vi "Add New Pos.vi"(0 "CS++Motor in":refnum<class "CS++Motor.lvclass">, 1 "Referenced":bool[](array[boolean]), 3 "MovementList In":T2(array[cluster]), 4 "NewPos-Data":T1, 5 "error in (no error)":errorcluster, 7 "LastPos In":cluster{dbl[]}[](array[cluster]), 8 "Axis Overwrite?":bool, 9 "AxisNumber":u8, 11 "ActPos":dbl[](array[numeric])) -> (13 "LastPos Out":cluster{dbl[]}[](array[cluster]), 14 "CS++Motor out":refnum<class "CS++Motor.lvclass">, 17 "MovementList Out":T2(array[cluster]), 19 "error out":errorcluster)   [LabVIEW 2016, in "CS++Motor.lvlib" / "CS++Motor.lvclass"]
doc: "This VI adds new position information to the Motor Base class actor. This information is written in a list and the commands are sent to the device once it is not busy."
uses:
  CS++Motor.lvclass
  PV-Enum-n.ctl
  CSPP_Core/Classes/CS++ProcessVariables/ProcessVariable/PV.lvclass
  CS++Motor.lvclass/CS++Motor.ctl
  CSPP_Core/Classes/CS++ProcessVariables/ProcessVariable/PV.lvclass/PV.ctl
  CSPP_Core/Classes/CS++ProcessVariables/ProcessVariable/Write Data.vi
  CSPP_Core/Classes/CS++ProcessVariables/ProcessVariable/Write Timestamp.vi
  CSPP_Core/Classes/CS++ProcessVariables/ProcessVariable/Write Quality.vi
  CSPP_Core/Classes/CS++ProcessVariables/ProcessVariable/Write status.vi
  CSPP_Core/Classes/CS++ProcessVariables/PVConnection/PVConnection.lvclass
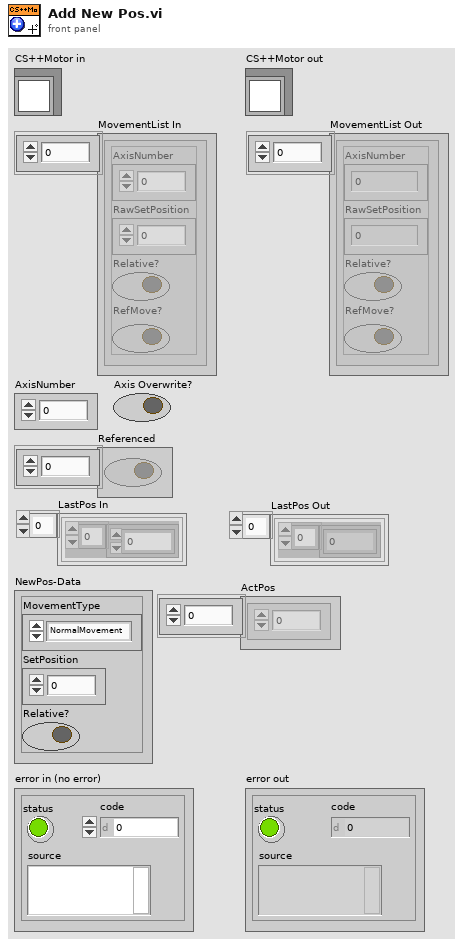
[diagram p1: front panel]
types:
  T1 = cluster{"MovementType":enum16{"NormalMovement", "ReferenceMovement", "StopMovement"}, "SetPosition":dbl, "Relative?":bool}
  T2 = cluster{"AxisNumber":u8, "RawSetPosition":dbl, "Relative?":bool, "RefMove?":bool}[]
  T3 = typedef "CS++Motor.lvlib/CS++Motor.lvclass/PV-Enum-n.ctl" = enum16{"PhysicalName", "unit", "ActPosition", "SetPosition", "RawSetPosition", "StartVelocity", "StopVelocity", "Acceleration", "RangeMin", "RangeMax", "Scaling", "ScalingOffset", "RangeRefError", "LogicalPositionArray", "NoOfCommands"}
  T4 = enum16{"NormalMovement", "ReferenceMovement", "StopMovement"}
  T5 = cluster{"AxisNumber":u8, "RawSetPosition":dbl, "Relative?":bool, "RefMove?":bool}
  T6 = cluster{"LogicalName":string, "PhysicalName":string, "unit":string, "Scaling":dbl, "Scaling Offset":dbl, "StartVelocity":dbl, "StopVelocity":dbl, "Acceleration":dbl, "RangeMin":dbl, "RangeMax":dbl, "LogicalPos-Array":cluster{"LogicalPosition":string, "SetPosition":dbl}[]}[]
  T7 = cluster{"LogicalName":string, "PhysicalName":string, "unit":string, "Scaling":dbl, "Scaling Offset":dbl, "StartVelocity":dbl, "StopVelocity":dbl, "Acceleration":dbl, "RangeMin":dbl, "RangeMax":dbl, "LogicalPos-Array":cluster{"LogicalPosition":string, "SetPosition":dbl}[]}
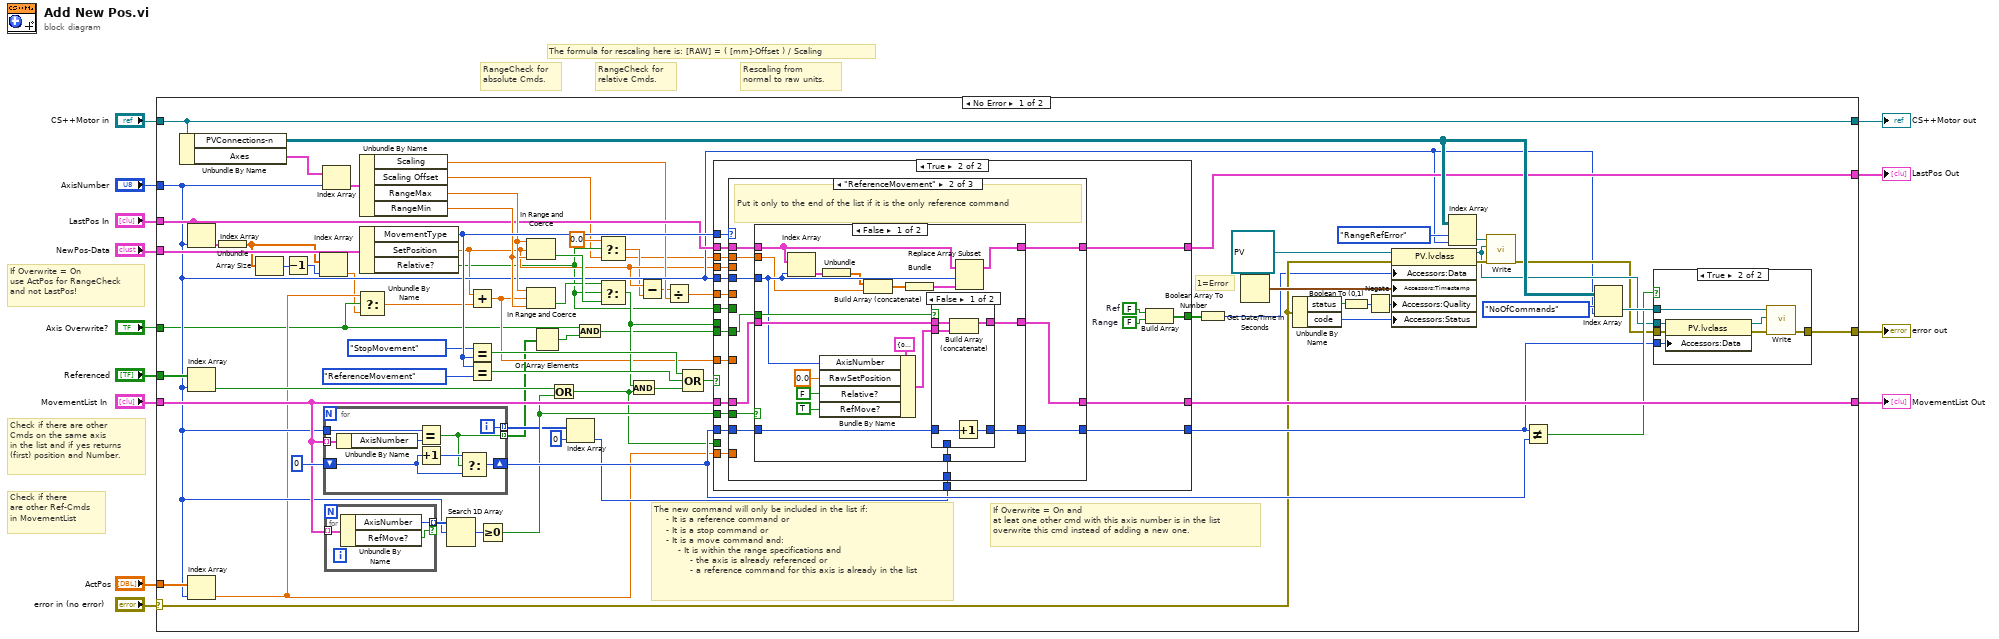
[diagram p0: block diagram]
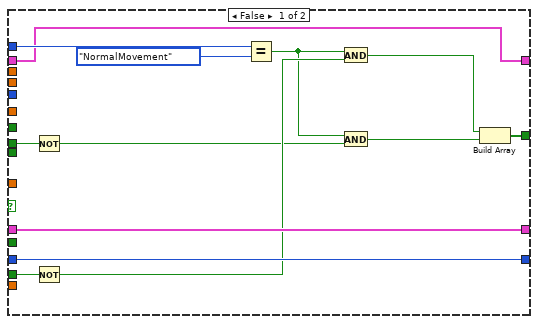
[diagram p2: hidden frame]
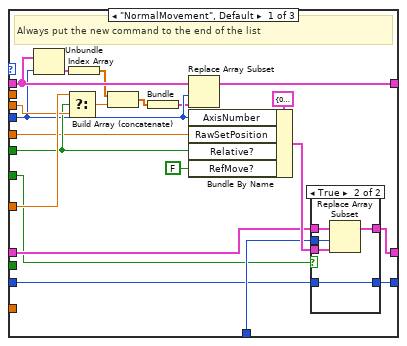
[diagram p3: hidden frame]
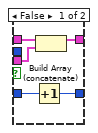
[diagram p4: hidden frame]
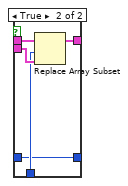
[diagram p5: hidden frame]
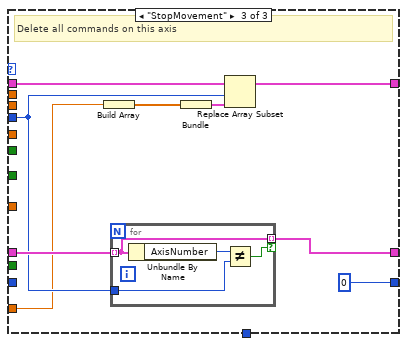
[diagram p7: hidden frame]
diagram:
  # "The formula for rescaling here is: [RAW] = ( [mm]-Offset ) / Scaling"
  # "Check if there are other\nCmds on the same axis \nin the list and if yes returns\n(first) position and Number."
  # "Check if there\nare other Ref-Cmds\nin MovementList"
  # "Rescaling from\nnormal to raw units."
  # "RangeCheck for\nrelative Cmds."
  # "RangeCheck for\nabsolute Cmds."
  # "If Overwrite = On\nuse ActPos for RangeCheck\nand not LastPos!"
  n1 = case shown="No Error" "error in (no error)" {
    selector: "error in (no error)" -> [w62 w228]
    tunnel: [w33 w228] -> w12
    tunnel: [w86 w227] -> w10
    tunnel: "CS++Motor in" -> [w86 w227]
    tunnel: "Referenced" -> [w81 _]
    tunnel: "NewPos-Data" -> [w83 _]
    tunnel: "MovementList In" -> [w70 w226]
    tunnel: "AxisNumber" -> [w29 _]
    tunnel: [w78 w226] -> w5
    tunnel: "LastPos In" -> [w40 _]
    tunnel: [w39 _] -> w1
    tunnel: "ActPos" -> [w38 _]
    tunnel: "Axis Overwrite?" -> [w26 _]
    frame No Error {
      # "If Overwrite = On and\nat leat one other cmd with this axis number is in the list\noverwrite this cmd instead of adding a new one."
      # "1=Error"
      # "The new command will only be included in the list if:\n    - It is a reference command or\n    - It is a stop command or\n    - It is a move command and:\n        - It is within the range specifications and\n            - the axis is already referenced or\n            - a reference command for this axis is already in the list"
      n2 = Unbundle By Name(w86) -> ("PVConnections-n"=w64:refnum<class "PVConnection.lvclass">[][], "Axes"=w85:T6)
      n3 = Index Array(array=w40, index=w29) -> (element=w18:cluster{dbl[]})
      n4 = Index Array(array=w81, index=w29) -> (element=w49:bool)
      n5 = Index Array(array=w38, index=w29) -> (element=w27:dbl)
      n6 = Unbundle(w18) -> (w16:dbl[])
      n7 = Array Size(array=w16) -> (size(s)=w15:i32)
      n8 = Decrement(x=w15) -> (x-1=w14:i32)
      n9 = Index Array(array=w16, index=w14) -> (element=w17:dbl)
      n10 = Index Array(array=w85, index=w29) -> (element=w84:T7)
      n11 = for {
        tunnel: w70 -> [w217] mode=indexing
        tunnel: w29 -> [w215]
        shift-right: [w214] -> w75
        shift-left: 0 -> [w212]
        tunnel: [w211] -> w36 mode=indexing if=w210
        tunnel: [w210] -> w32 mode=indexing
        i -> [w211]
        n12 = Unbundle By Name(w217) -> ("AxisNumber"=w216:u8)
        n13 = Equal?(x=w215, y=w216) -> (x = y?=w210:bool)
        n14 = Increment(x=w212) -> (x+1=w213:i32)
        n15 = Select(t=w213, s=w210, f=w212) -> (s? t:f=w214:i32)
      }
      n16 = for {
        tunnel: w70 -> [w209] mode=indexing
        tunnel: [w208] -> w72 mode=indexing if=w207
        n17 = Unbundle By Name(w209) -> ("AxisNumber"=w208:u8, "RefMove?"=w207:bool)
      }
      n18 = Select(t=w27, s=w26, f=w17) -> (s? t:f=w28:dbl)
      n19 = Unbundle By Name(w84) -> ("Scaling"=w25:dbl, "Scaling Offset"=w19:dbl, "RangeMax"=w42:dbl, "RangeMin"=w41:dbl)
      n20 = Unbundle By Name(w83) -> ("MovementType"=w68:T4, "SetPosition"=w24:dbl, "Relative?"=w22:bool)
      n21 = Search 1D Array(1D array=w72, element=w29) -> (index of element=w71:i32)  [unwired: 1 in]
      n22 = Add(x=w24, y=w28) -> (x+y=w37:dbl)
      n23 = Equal?(x=T4."StopMovement" ("y"), y=w68) -> (x = y?=w65:bool)
      n24 = Equal?(x=w68, y=T4."ReferenceMovement") -> (x = y?=w66:bool)
      n25 = Greater Or Equal To 0?(x=w71) -> (x >= 0?=w69:bool)
      n26 = In Range and Coerce(upper limit=w42, x=w24, lower limit=w41) -> (In Range?=w45:bool)  [unwired: 1 out]
      n27 = In Range and Coerce(upper limit=w42, x=w37, lower limit=w41) -> (In Range?=w43:bool)  [unwired: 1 out]
      n28 = Or Array Elements(Boolean array=w32) -> (logical OR=w31:bool)
      n29 = Or(x=w49, y=w69) -> (x .or. y?=w48:bool)
      n30 = Index Array(array=w36, index=0) -> (element=w34:i32)
      n31 = And(x=w26, y=w31) -> (x .and. y?=w30:bool)
      n32 = Select(t=0.0, s=w22, f=w19) -> (s? t:f=w21:dbl)
      n33 = Select(t=w43, s=w22, f=w45) -> (s? t:f=w44:bool)
      n34 = And(x=w44, y=w48) -> (x .and. y?=w50:bool)
      n35 = Subtract(x=w24, y=w21) -> (x-y=w23:dbl)
      n36 = Divide(x=w23, y=w25) -> (x/y=w82:dbl)
      n37 = Compound Arithmetic op=OR(w65, w66, w50) -> (w53:bool)
      n38 = case shown="True" w53 {
        tunnel: w22 -> [_ w119]
        tunnel: w82 -> [_ w118]
        tunnel: [w99 w117] -> w78
        tunnel: w75 -> [w98 w116]
        tunnel: [w98 w115] -> w74
        tunnel: w70 -> [w99 w114]
        tunnel: w69 -> [_ w113]
        tunnel: w68 -> [w96 w112]
        tunnel: w29 -> [_ w111]
        tunnel: [w97 w108] -> w51
        tunnel: w48 -> [w93 _]
        tunnel: w44 -> [w89 _]
        tunnel: w40 -> [w87 w107]
        tunnel: [w87 w106] -> w39
        tunnel: w37 -> [_ w105]
        tunnel: w27 -> [_ w104]
        tunnel: w24 -> [_ w103]
        tunnel: w30 -> [_ w102]
        tunnel: w34 -> [_ w101]
        tunnel: w19 -> [_ w100]
        frame False {
          n39 = Not(x=w89) -> (.not. x?=w88:bool)
          n40 = Not(x=w93) -> (.not. x?=w92:bool)
          n41 = Equal?(x=w96, y=T4."NormalMovement") -> (x = y?=w91:bool)
          n42 = And(x=w91, y=w92) -> (x .and. y?=w94:bool)
          n43 = And(x=w91, y=w88) -> (x .and. y?=w90:bool)
          n44 = Build Array(w94, w90) -> (w97:bool[])
        }
        frame True {
          w110 = FALSE  # Range
          w109 = FALSE  # Ref
          n45 = case shown="\"ReferenceMovement\"" w112 {
            tunnel: w114 -> [w136 w161 w202]
            tunnel: [w137 w160 w201] -> w117
            tunnel: w111 -> [w125 w159 w197]
            tunnel: w119 -> [w132 _ _]
            tunnel: w118 -> [w131 _ _]
            tunnel: w116 -> [w127 w157 _]
            tunnel: [w128 w158 0] -> w115
            tunnel: w113 -> [_ w156 _]
            tunnel: w107 -> [w126 w155 w199]
            tunnel: [w135 w154 w198] -> w106
            tunnel: w105 -> [w134 _ _]
            tunnel: w104 -> [_ _ w196]
            tunnel: w103 -> [w133 _ _]
            tunnel: w102 -> [w129 w153 _]
            tunnel: w101 -> [w130 w152 _]
            tunnel: w100 -> [_ w151 _]
            frame "NormalMovement", Default {
              # "Always put the new command to the end of the list"
              n46 = Index Array(array=w126, index=w125) -> (element=w124:cluster{dbl[]})
              n47 = Select(t=w134, s=w132, f=w133) -> (s? t:f=w122:dbl)
              n48 = Unbundle(w124) -> (w123:dbl[])
              n49 = Build Array (concatenate)(w123, w122) -> (w121:dbl[])
              n50 = Bundle(w121) -> (w120:cluster{dbl[]})  [unwired: 1 in]
              n51 = Replace Array Subset(array=w126, new element=w120, index=w125) -> (w135:cluster{dbl[]}[])
              n52 = Bundle By Name(cluster=T5 {"AxisNumber"=0, "RawSetPosition"=0.0, "Relative?"=FALSE, "RefMove?"=FALSE} ("SingleMovement"), "AxisNumber"=w125, "RawSetPosition"=w131, "Relative?"=w132, "RefMove?"=FALSE) -> (w138:T5)
              n53 = case shown="True" w129 {
                tunnel: w138 -> [w145 w148]
                tunnel: [w144 w149] -> w137
                tunnel: w136 -> [w143 w150]
                tunnel: w130 -> [_ w147]
                tunnel: [w141 w146] -> w128
                tunnel: w127 -> [w142 w146]
                frame False {
                  n54 = Increment(x=w142) -> (x+1=w141:i32)
                  n55 = Build Array (concatenate)(w143, w145) -> (w144:T2)
                }
                frame True {
                  n56 = Replace Array Subset(array=w150, new element=w148, index=w147) -> (w149:T2)
                }
              }
            }
            frame "ReferenceMovement" {
              # "Put it only to the end of the list if it is the only reference command"
              n57 = case shown="False" w156 {
                tunnel: [w180 w193] -> w160
                tunnel: w161 -> [w176 w193]
                tunnel: w159 -> [w166 _]
                tunnel: [w169 w192] -> w158
                tunnel: w157 -> [w170 w192]
                tunnel: w155 -> [w167 w191]
                tunnel: [w173 w191] -> w154
                tunnel: w153 -> [w172 _]
                tunnel: w152 -> [w171 _]
                tunnel: w151 -> [w164 _]
                frame False {
                  n58 = Index Array(array=w167, index=w166) -> (element=w168:cluster{dbl[]})
                  n59 = Bundle By Name(cluster=T5 {"AxisNumber"=0, "RawSetPosition"=0.0, "Relative?"=FALSE, "RefMove?"=FALSE} ("SingleMovement"), "AxisNumber"=w166, "RawSetPosition"=0.0 ("RawActPosition"), "Relative?"=FALSE, "RefMove?"=TRUE) -> (w175:T5)
                  n60 = Unbundle(w168) -> (w165:dbl[])
                  n61 = Build Array (concatenate)(w165, w164) -> (w163:dbl[])
                  n62 = Bundle(w163) -> (w162:cluster{dbl[]})  [unwired: 1 in]
                  n63 = case shown="False" w172 {
                    tunnel: [w185 w189] -> w180
                    tunnel: w176 -> [w184 w190]
                    tunnel: w175 -> [w183 w188]
                    tunnel: w171 -> [_ w187]
                    tunnel: w170 -> [w182 w186]
                    tunnel: [w181 w186] -> w169
                    frame False {
                      n64 = Build Array (concatenate)(w184, w183) -> (w185:T2)
                      n65 = Increment(x=w182) -> (x+1=w181:i32)
                    }
                    frame True {
                      n66 = Replace Array Subset(array=w190, new element=w188, index=w187) -> (w189:T2)
                    }
                  }
                  n67 = Replace Array Subset(array=w167, new element=w162, index=w166) -> (w173:cluster{dbl[]}[])
                }
                frame True {
                }
              }
            }
            frame "StopMovement" {
              # "Delete all commands on this axis"
              n68 = Build Array(w196) -> (w195:dbl[])
              n69 = for {
                tunnel: w202 -> [w204] mode=indexing
                tunnel: w197 -> [w205]
                tunnel: [w204] -> w201 mode=indexing if=w203
                n70 = Unbundle By Name(w204) -> ("AxisNumber"=w206:u8)
                n71 = Not Equal?(x=w206, y=w205) -> (x != y?=w203:bool)
              }
              n72 = Bundle(w195) -> (w194:cluster{dbl[]})  [unwired: 1 in]
              n73 = Replace Array Subset(array=w199, new element=w194, index=w197) -> (w198:cluster{dbl[]}[])
            }
          }
          n74 = Build Array(w109, w110) -> (w108:bool[])
        }
      }
      n75 = Boolean Array To Number(Boolean array=w51) -> (number=w52:u32)
      n76 = Get Date/Time In Seconds() -> (seconds since 1Jan1904=w63:timestamp)
      n77 = Unbundle By Name(w62) -> ("status"=w56:bool, "code"=w59:i32)
      n78 = Boolean To (0,1)(Boolean=w56) -> (0, 1=w58:i16)
      n79 = Negate(x=w58) -> (-x=w57:i16)
      n80 = property class="PV.lvclass"(reference=refnum<class "PV.lvclass"> refnum ("PV"), error in=w62, "Accessors:Data"=w52, "Accessors:Timestamp"=w63, "Accessors:Quality"=w57, "Accessors:Status"=w59) -> (reference out=w47:refnum<class "PV.lvclass">, error out=w55:errorcluster)
      n81 = Index Array(array=w64, index (row)=PV-Enum-n."RangeRefError" ("PV-Enum-n"), index (col)=w29) -> (element=w54:refnum<class "PVConnection.lvclass">)
      n82 = call "Write.vi"("error in (no error)"=w55, "PV"=w47, "PVConnection in"=w54) -> ("error out"=w46:errorcluster)  [unwired: 7 in, 1 out]
      n83 = Not Equal?(x=w74, y=w75) -> (x != y?=w77:bool)
      n84 = Index Array(array=w64, index (row)=PV-Enum-n."NoOfCommands" ("PV-Enum-n"), index (col)=w29) -> (element=w79:refnum<class "PVConnection.lvclass">)
      n85 = case shown="True" w77 {
        tunnel: w46 -> [w218 w225]
        tunnel: w47 -> [_ w224]
        tunnel: w79 -> [_ w221]
        tunnel: [w218 w220] -> w33
        tunnel: w74 -> [_ w219]
        frame False {
        }
        frame True {
          n86 = property class="PV.lvclass"(reference=w224, error in=w225, "Accessors:Data"=w219) -> (reference out=w222:refnum<class "PV.lvclass">, error out=w223:errorcluster)
          n87 = call "Write.vi"("error in (no error)"=w223, "PV"=w222, "PVConnection in"=w221) -> ("error out"=w220:errorcluster)  [unwired: 7 in, 1 out]
        }
      }
    }
    frame Error {
    }
  }
  "error out" <- w12
  "CS++Motor out" <- w10
  "MovementList Out" <- w5
  "LastPos Out" <- w1
